vi "Number of Address Map Elements.vi"(2 "niUSRP Rx Core v1 FPGA":refnum<class "niUSRP Tx Core v1 FPGA.lvclass">) -> (6 "number of elements":u8)   [LabVIEW 2025, in "niUSRP Tx Core v1 FPGA.lvclass"]
uses:
  niUSRP Tx Core v1 FPGA.lvclass
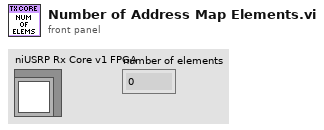
[diagram p1: front panel]
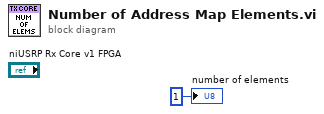
[diagram p0: block diagram]
diagram:
  "number of elements" <- u8 1 ("number of elements")
